vi "Write Root.vi"(8 "Error In":errorcluster, 10 "Root":path=path "", 11 "File In":refnum<class "File.lvclass">) -> (0 "Error Out":errorcluster, 3 "File Out":refnum<class "File.lvclass">)   [LabVIEW 2018, in "Toolkit.lvlib" / "Loaders.lvlib" / "File.lvclass"]
uses:
  File.lvclass
  File.lvclass/File.ctl
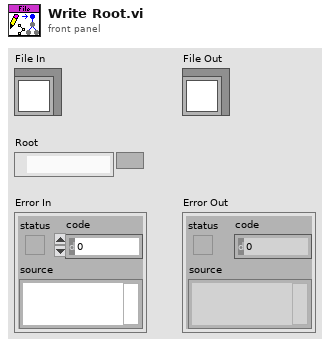
[diagram p1: front panel]
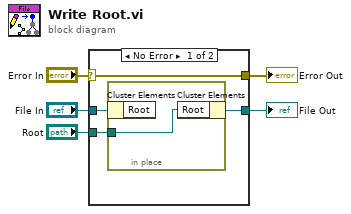
[diagram p0: block diagram]
diagram:
  n1 = case shown="No Error" "Error In" {
    selector: "Error In" -> [w9 w11]
    tunnel: [w9 w11] -> w4
    tunnel: [w6 w12] -> w2
    tunnel: "File In" -> [w8 w12]
    tunnel: "Root" -> [w7 _]
    frame No Error {
      n2 = in-place {
        in-place-border: w7 -> [w10]
        n3 = in-place-cluster #1(w8) -> ()  [unwired: 1 out]
        n4 = in-place-cluster #1("Root"=w10) -> (w6:refnum<class "File.lvclass">)
      }
    }
    frame Error {
    }
  }
  "Error Out" <- w4
  "File Out" <- w2
